vi "Template Pattern - Caller.vi"(4 "Message Size":T2 {"Message Width" min=-1 step=1; "Message Height" min=-1 step=1}, 6 "Theme":refnum<class "Theme.lvclass">, 7 "standard":T1="info", 8 "error in (no error)":errorcluster, 9 "Graphic":path, 10 "Message":string, 11 "Pop-Up in":refnum<class "PNG Parent.lvclass">) -> (0 "error out":errorcluster, 3 "Pop-Up out":refnum<class "PNG Parent.lvclass">)   [LabVIEW 2021, in "Pop-Up.lvlib" / "PNG Parent.lvclass"]
doc: "The TEMPLATE PATTERN OOP VI will define the way that the Display function will be called in the PNG type pop-up class. \n\n<b>Code Developed By:</b> +\nDaniel Coons +\nhttps://github.com/danielcoons/tsc-pop-up"
uses:
  PNG Parent.lvclass
  C:/Development/Open Source/tsc-pop-up/Popup/Popup.lvclass
  Theme/Theme.lvclass
  Popup/message info--typedef.ctl
  Graphics.ctl
  Popup/Popup.lvclass/Popup.ctl
  Popup/Data Member Access/Read Theme.vi
  Popup/Data Member Access/Write Theme.vi
  Popup/Data Member Access/Write Pic Width.vi
  Popup/Data Member Access/Write Pic Height.vi
  Popup/Data Member Access/Write Message Size.vi
  PNG Parent.lvclass/PNG Parent.ctl
  Popup/Popup.lvclass
  Pop-Up.lvlib
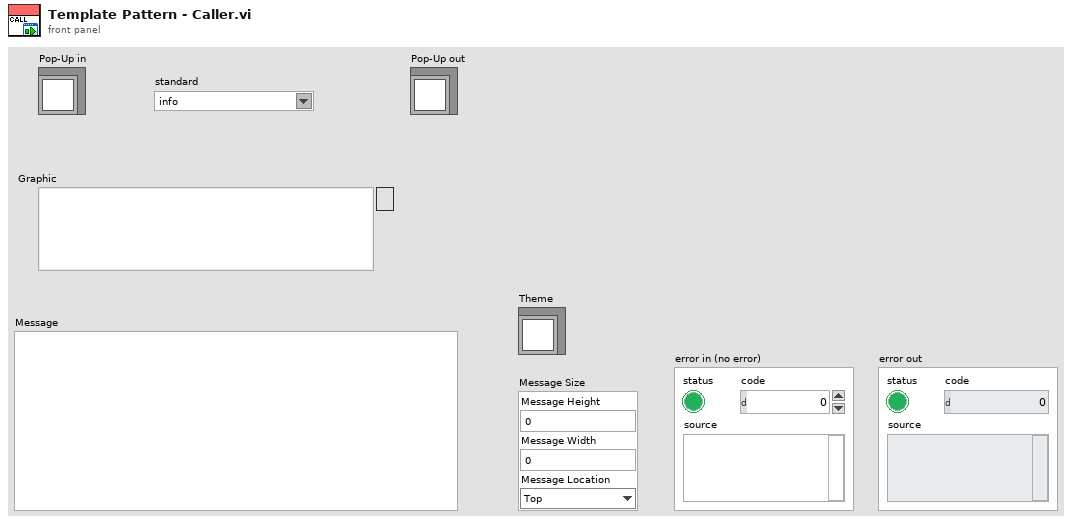
[diagram p1: front panel]
types:
  T1 = typedef "Pop-Up.lvlib/Graphics.ctl" = string
  T2 = typedef "Pop-Up.lvlib/Popup.lvclass/message info--typedef.ctl" = cluster{"Message Height":i32, "Message Width":i32, "Message Location":enum16{"Top", "Bottom", "Right", "Left"}}
  T3 = typedef "imagedata.ctl" = cluster{"image type":i32, "image depth":i32, "image":u8[], "mask":u8[], "colors":u32[], "Rectangle":cluster{"left":i16, "top":i16, "right":i16, "bottom":i16}}
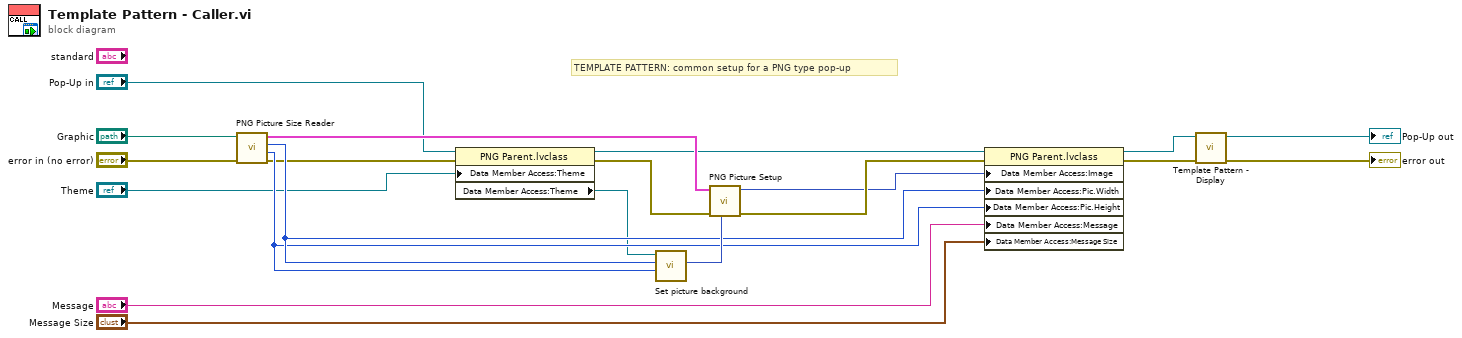
[diagram p0: block diagram]
diagram:
  # "TEMPLATE PATTERN: common setup for a PNG type pop-up"
  n1 = call "PNG Picture Size Reader.vi"("error in (no error)"="error in (no error)", "Graphic"="Graphic") -> ("error out"=w14:errorcluster, "pic height"=w15:i16, "pic width"=w16:i16, "custom image"=w17:T3)  [unwired: 6 in]
  n2 = property class="PNG Parent.lvclass"(reference="Pop-Up in", error in=w14, "Data Member Access:Theme"="Theme") -> (reference out=w5:refnum<class "PNG Parent.lvclass">, error out=w13:errorcluster, "Data Member Access:Theme"=w12:refnum<class "Theme.lvclass">)
  n3 = call "Set picture background.vi"("pic height"=w15, "pic width"=w16, "Theme in"=w12) -> ("background"=w18:picture)  [unwired: 6 in, 2 out]
  n4 = call "PNG Picture Setup.vi"("picture background"=w18, "error in (no error)"=w13, "image data"=w17) -> ("error out"=w20:errorcluster, "picture"=w19:picture)  [unwired: 7 in]
  n5 = property class="PNG Parent.lvclass"(reference=w5, error in=w20, "Data Member Access:Image"=w19, "Data Member Access:Pic.Width"=w16, "Data Member Access:Pic.Height"=w15, "Data Member Access:Message"="Message", "Data Member Access:Message Size"="Message Size") -> (reference out=w2:refnum<class "PNG Parent.lvclass">, error out=w4:errorcluster)
  n6 = call "Template Pattern - Display.vi"("error in (no error)"=w4, "PopUp in"=w2) -> ("error out"=→"error out":errorcluster, "PopUp out"=→"Pop-Up out":refnum<class "PNG Parent.lvclass">)  [unwired: 8 in]
